vi "Append.vi"(6 "Append":string, 9 "Rename Suffix":string, 10 "Name Suffix":string) -> (1 "Post":string, 2 "Pre":string)   [LabVIEW 2020, in "_Rename.lvlib" / "_Rename.lvclass"]
uses:
  _Rename.lvclass
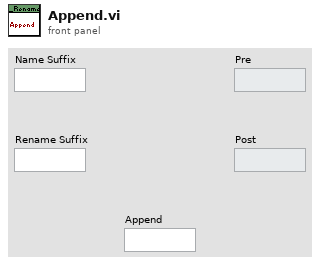
[diagram p1: front panel]
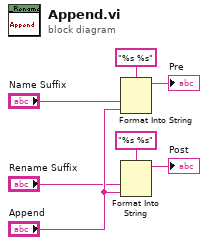
[diagram p0: block diagram]
diagram:
  n1 = Format Into String(format string="%s %s", "Name Suffix", "Append") -> (resulting string=→"Pre":string)  [unwired: 2 in, 1 out]
  n2 = Format Into String(format string="%s %s", "Rename Suffix", "Append") -> (resulting string=→"Post":string)  [unwired: 2 in, 1 out]
